vi "get_all_lm_fits.vi"(8 "Error In":errorcluster, 10 "Sample":string, 11 "File Path":path) -> (0 "Error Out":errorcluster)   [LabVIEW 2019]
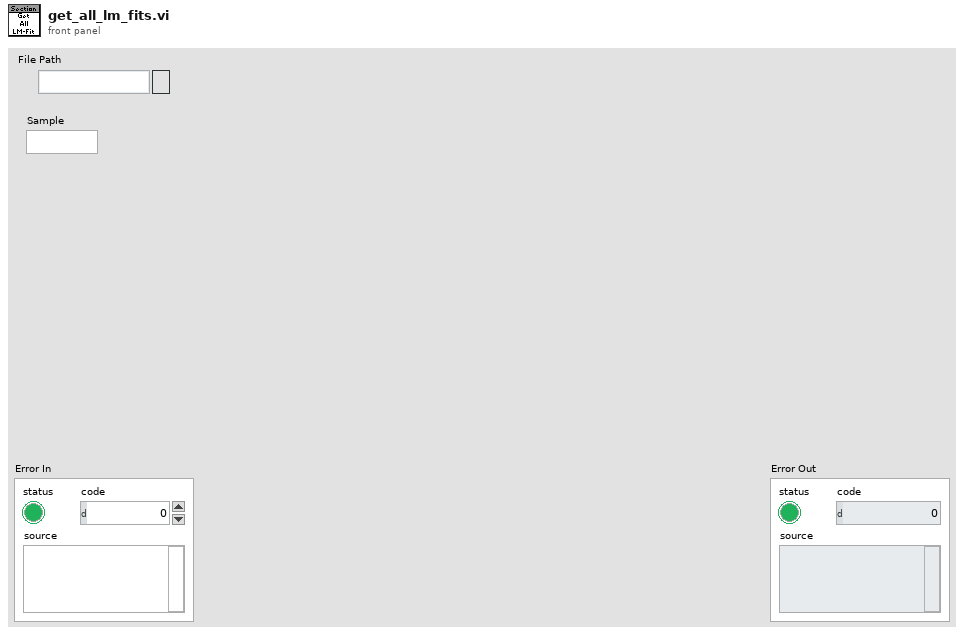
[diagram p1: front panel]
types:
  T1 = typedef "sample_results_cluster_typedef.ctl" = cluster{"File Path":string, "Sample":string, "Threshold":dbl, "Parameters":T2, "Writeable Parameters":T3, "Gain Results":T4[]}
  T2 = typedef "parameters_cluster_typedef.ctl" = cluster{"m1":dbl, "m2":dbl, "m3":dbl, "c":dbl, "D":dbl, "Beta":dbl, "center x":dbl, "center y":dbl}
  T3 = typedef "writeable_section_parameters_cluster_typedef.ctl" = cluster{"Section":string, "Method":i32, "Edge Mode":i32, "Grid Constant":i32, "Manual Sequence":i32, "ROI Size":i32, "Min Grain Size":dbl, "Comments":string, "File Path":string}
  T4 = typedef "grain_results_cluster_typedef.ctl" = cluster{"Grain Number":i32, "xi":dbl[], "phiin":dbl[], "Intensity":dbl[][], "Best Fit Intensity":dbl[][], "Best Fit Parameters":dbl[][], "Polarizer 1 Angle":dbl[][], "Polarizer 2 Angle":dbl[][], "Best Extinction Angle":dbl[], "Best Extinction Angle Corrected":dbl[], "Thetac":dbl, "Phic":dbl, "ROI":cluster{"Global Rectangle":i32[], "Contours":cluster{"Contour Type":u32, "ROI Type":u32, "Points":i32[]}[]}, "a":dbl, "b":dbl, "sequences available":dbl, "sequences used":dbl, "Contrast":dbl[], "Rsq":dbl}
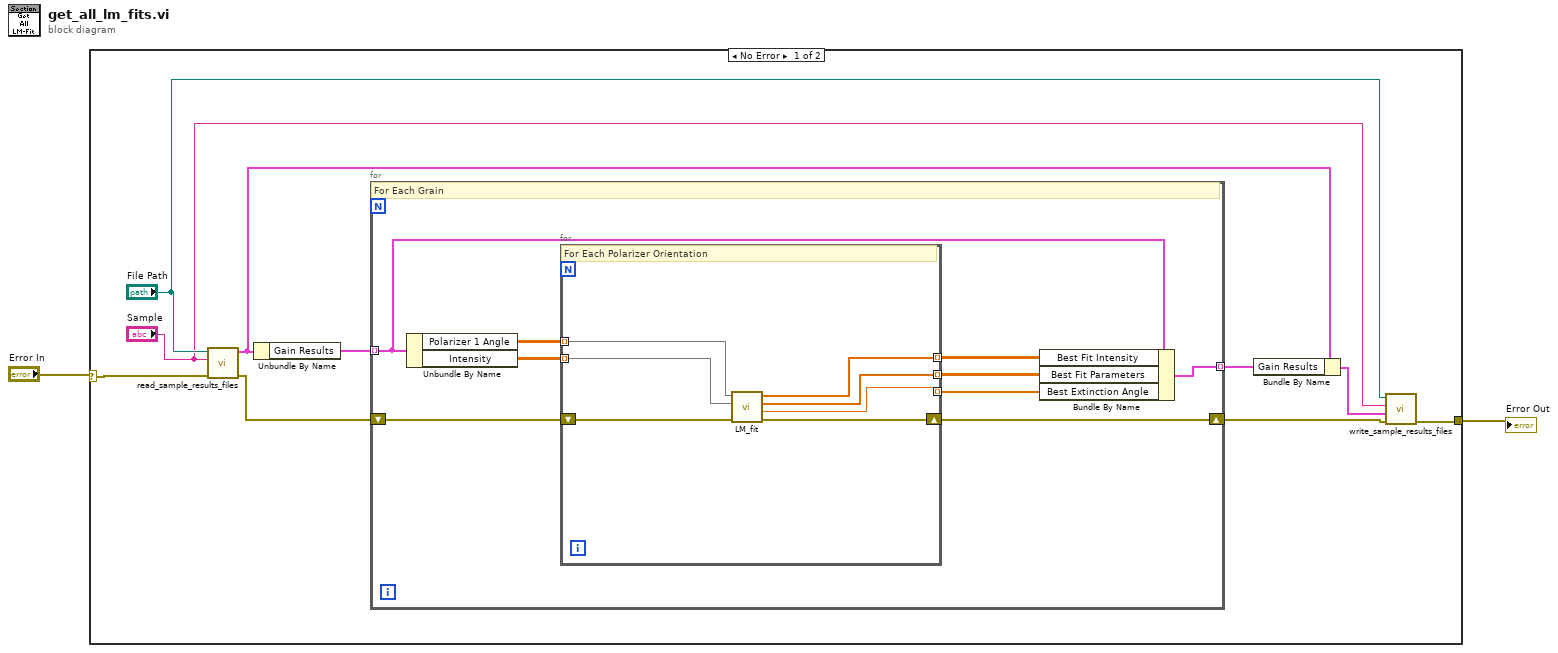
[diagram p0: block diagram]
diagram:
  n1 = case shown="No Error" "Error In" {
    selector: "Error In" -> [w12 w29]
    tunnel: [w3 w29] -> w1
    frame No Error {
      n2 = call "read_sample_results_files.vi"("Error In"=w12, "Sample"="Sample", "File Path"="File Path") -> ("Error Out"=w10:errorcluster, "Sample Results"=w9:T1)  [unwired: 7 in]
      n3 = Unbundle By Name(w9) -> ("Gain Results"=w11:T4[])
      n4 = for {
        tunnel: w11 -> [w18] mode=indexing
        shift-right: [w14] -> w7
        shift-left: w10 -> [w19]
        tunnel: [w15] -> w8 mode=indexing
        # "For Each Grain"
        n5 = Unbundle By Name(w18) -> ("Polarizer 1 Angle"=w21:dbl[][], "Intensity"=w20:dbl[][])
        n6 = for {
          tunnel: w21 -> [w28] mode=indexing
          tunnel: w20 -> [w27] mode=indexing
          shift-right: [w25] -> w14
          shift-left: w19 -> [w26]
          tunnel: [w24] -> w16 mode=indexing
          tunnel: [w23] -> w17 mode=indexing
          tunnel: [w22] -> w13 mode=indexing
          # "For Each Polarizer Orientation"
          n7 = call "LM_fit.vi"("Error In"=w26, "Intensities"=w27, "Angles"=w28) -> ("Error Out"=w25:errorcluster, "Extinction Angle"=w22:dbl, "best fit parameters"=w23:dbl[], "best nonlinear fit"=w24:dbl[])  [unwired: 5 in]
        }
        n8 = Bundle By Name(cluster=w18, "Best Fit Intensity"=w16, "Best Fit Parameters"=w17, "Best Extinction Angle"=w13) -> (w15:T4)
      }
      n9 = Bundle By Name(cluster=w9, "Gain Results"=w8) -> (w4:T1)
      n10 = call "write_sample_results_files.vi"("Error In"=w7, "Sample Results"=w4, "Sample"="Sample", "File Path"="File Path") -> ("Error Out"=w3:errorcluster)  [unwired: 7 in]
    }
    frame Error {
    }
  }
  "Error Out" <- w1
